vi "Climb Switches.vi"(11 "Enum":enum16{"Start", "Run", "End"}(ring)) -> (3 "Limit Values":T1)   [LabVIEW 2012]
uses:
  TypeDefs/Digital Module 1.ctl
  <vilib>/Rock Robotics/SystemInterfaces/Typedef/FPGA_TypedefDigitalModule.ctl
  <vilib>/Rock Robotics/SystemInterfaces/DIO/FPGA_DIOChannel.ctl
panel:
  in  "Digital Module A":T2={"Module"=enum."Digital Module 1", "Unassigned"=enum."DIO 1", "Unassigned"=enum."DIO 2", "Unassigned"=enum."DIO 3", "Unassigned"=enum."DIO 4", "Unassigned"=enum."DIO 5", "Unassigned"=enum."DIO 6", "Unassigned"=enum."DIO 7", "Unassigned"=enum."DIO 8", "Unassigned"=enum."DIO 9", "Unassigned"=enum."DIO 10", "Unassigned"=enum."DIO 11", "Unassigned"=enum."DIO 12", "Unassigned"=enum."DIO 13", "Unassigned"=enum."DIO 14"}
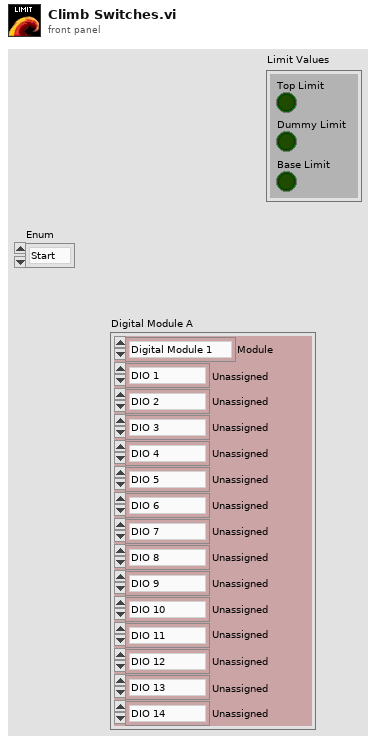
[diagram p1: front panel]
types:
  T1 = cluster{"Top Limit":bool, "Dummy Limit":bool, "Base Limit":bool}
  T2 = typedef "Digital Module 1.ctl" = cluster{"Module":T3, "Unassigned":T4, "Unassigned":T4, "Unassigned":T4, "Unassigned":T4, "Unassigned":T4, "Unassigned":T4, "Unassigned":T4, "Unassigned":T4, "Unassigned":T4, "Unassigned":T4, "Unassigned":T4, "Unassigned":T4, "Unassigned":T4, "Unassigned":T4}
  T3 = typedef "FPGA_TypedefDigitalModule.ctl" = enum16{"Digital Module 1", "Digital Module 2"}
  T4 = typedef "FPGA_DIOChannel.ctl" = enum8{"DIO 1", "DIO 2", "DIO 3", "DIO 4", "DIO 5", "DIO 6", "DIO 7", "DIO 8", "DIO 9", "DIO 10", "DIO 11", "DIO 12", "DIO 13", "DIO 14", "Invalid"}
  T5 = typedef "WPI_DigitalInputDevRef.ctl" = cluster{"DevStatus":errorcluster, "DIO Channel":T4, "Digital Module":T3}
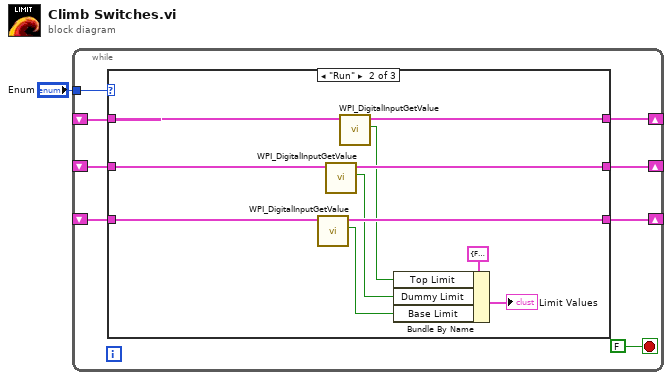
[diagram p0: block diagram]
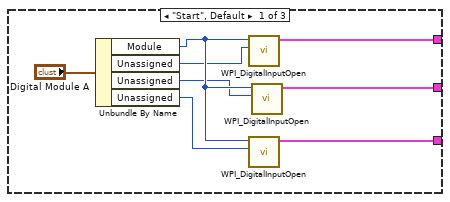
[diagram p2: hidden frame]
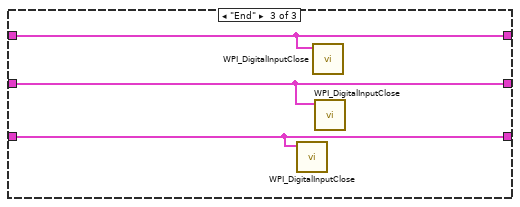
[diagram p3: hidden frame]
diagram:
  n1 = while {
    tunnel: "Enum" -> [w6]
    shift-right: [w8] -> _
    shift-left: _ -> [w7]
    shift-right: [w5] -> _
    shift-left: _ -> [w2]
    shift-right: [w4] -> _
    shift-left: _ -> [w3]
    stop <- FALSE stop-if-true
    n2 = case shown="\"Run\"" w6 {
      tunnel: [w17 w27 w31] -> w8
      tunnel: w7 -> [_ w28 w31]
      tunnel: [w11 w26 w30] -> w5
      tunnel: [w10 w23 w29] -> w4
      tunnel: w3 -> [_ w24 w29]
      tunnel: w2 -> [_ w25 w30]
      frame "Start", Default {
        n3 = Unbundle By Name("Digital Module A") -> ("Module"=w15:T3, "Unassigned"=w14:T4, "Unassigned"=w13:T4, "Unassigned"=w12:T4)
        n4 = call <vilib>:"WPI_DigitalInputOpen.vi"("DIO Channel"=w14, "Digital Module (Module 1)"=w15) -> ("DigitalInputDevRef"=w17:T5)  [unwired: 8 in, 1 out]
        n5 = call <vilib>:"WPI_DigitalInputOpen.vi"("DIO Channel"=w12, "Digital Module (Module 1)"=w15) -> ("DigitalInputDevRef"=w10:T5)  [unwired: 8 in, 1 out]
        n6 = call <vilib>:"WPI_DigitalInputOpen.vi"("DIO Channel"=w13, "Digital Module (Module 1)"=w15) -> ("DigitalInputDevRef"=w11:T5)  [unwired: 8 in, 1 out]
      }
      frame "Run" {
        n7 = call <vilib>:"WPI_DigitalInputGetValue.vi"("DigitalInputDevRef"=w24) -> ("Value"=w19:bool, "DigitalInputDevRef"=w23:T5)  [unwired: 8 in, 1 out]
        n8 = call <vilib>:"WPI_DigitalInputGetValue.vi"("DigitalInputDevRef"=w25) -> ("Value"=w20:bool, "DigitalInputDevRef"=w26:T5)  [unwired: 8 in, 1 out]
        n9 = call <vilib>:"WPI_DigitalInputGetValue.vi"("DigitalInputDevRef"=w28) -> ("Value"=w21:bool, "DigitalInputDevRef"=w27:T5)  [unwired: 8 in, 1 out]
        n10 = Bundle By Name(cluster=T1 {"Top Limit"=FALSE, "Dummy Limit"=FALSE, "Base Limit"=FALSE} ("Limit Values"), "Top Limit"=w21, "Dummy Limit"=w20, "Base Limit"=w19) -> (→"Limit Values":T1)
      }
      frame "End" {
        n11 = call <vilib>:"WPI_DigitalInputClose.vi"("DigitalInputDevRef"=w29) -> ()  [unwired: 10 in, 1 out]
        n12 = call <vilib>:"WPI_DigitalInputClose.vi"("DigitalInputDevRef"=w31) -> ()  [unwired: 10 in, 1 out]
        n13 = call <vilib>:"WPI_DigitalInputClose.vi"("DigitalInputDevRef"=w30) -> ()  [unwired: 10 in, 1 out]
      }
    }
  }
